vi "Test Resume Refreshing Trigger Broadcast.vi"(8 "error in (no error)":errorcluster, 11 "Test Case In":refnum<class "Debugger Test.lvclass">) -> (0 "error out":errorcluster, 3 "Test Case Out":refnum<class "Debugger Test.lvclass">)   [LabVIEW 2020, in "Debugger Test.lvclass"]
uses:
  Debugger Test.lvclass
  Debugger Test.lvclass/Debugger Test.ctl
  01074fa8-ee8a-411d-bc8b-fc92c4f90959.vi
  source/Process/Debug Process.lvclass
  source/Debugger/Debugger.lvclass
  C:/Git/astemes-triarc-debugger/source/Process/Debug Process.lvclass
  C:/Git/astemes-triarc-debugger/source/Debugger/Debugger.lvclass
  C:/Git/astemes-triarc-debugger/source/Debug Data Event/Debug Data Listener.lvclass
  <vilib>/Astemes/Triarc Framework/Broadcast Event Helpers/Broadcast Event Helpers.lvlib
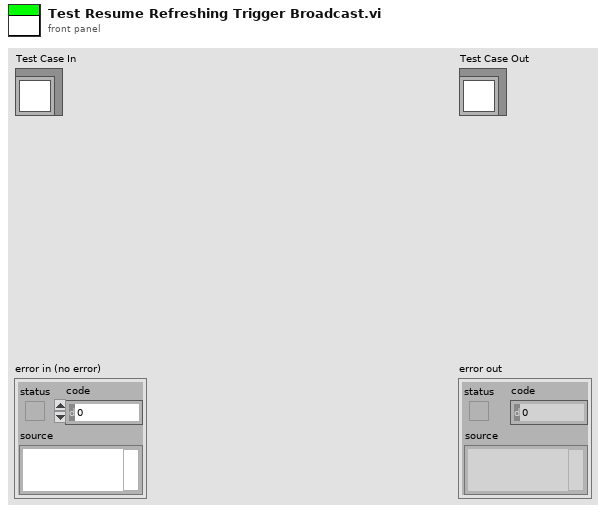
[diagram p1: front panel]
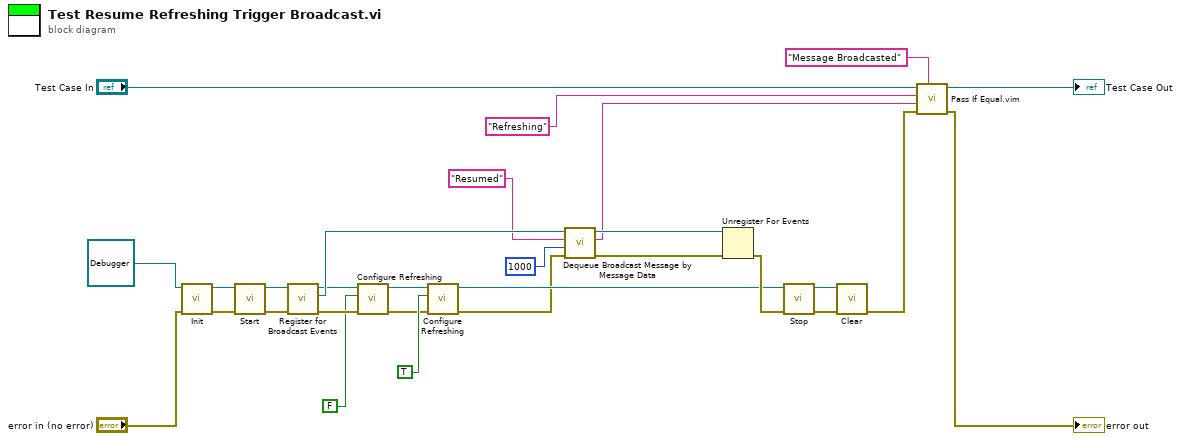
[diagram p0: block diagram]
diagram:
  n1 = call-dynamic "Init.vi"("error in (no error)"="error in (no error)", "Process In"=refnum<class "Debugger.lvclass"> refnum ("Debug Data Event In 2")) -> ("error out"=w25:errorcluster, "Process Out"=w26:refnum<class "Debugger.lvclass">)  [unwired: 8 in]
  n2 = call "Start.vi"("error in (no error)"=w25, "Process In"=w26) -> ("error out"=w23:errorcluster, "Process Out"=w24:refnum<class "Debugger.lvclass">)  [unwired: 7 in, 1 out]
  n3 = call "Register for Broadcast Events.vi"("error in (no error)"=w23, "Process In"=w24) -> ("error out"=w15:errorcluster, "Event Registration Refnum Out"=w16:refnum<event-registration>, "Process Out"=w6:refnum<class "Debugger.lvclass">)  [unwired: 7 in]
  n4 = call "Configure Refreshing.vi"("error in (no error)"=w15, "Refresh?"=FALSE, "Debugger In"=w6) -> ("error out"=w7:errorcluster, "Debugger Out"=w5:refnum<class "Debugger.lvclass">)  [unwired: 7 in]
  n5 = call "Configure Refreshing.vi"("error in (no error)"=w7, "Refresh?"=TRUE ("Show Send?"), "Debugger In"=w5) -> ("error out"=w8:errorcluster, "Debugger Out"=w9:refnum<class "Debugger.lvclass">)  [unwired: 7 in]
  n6 = call <vilib>:"Dequeue Broadcast Message by Message Data.vi"("error in (no error)"=w8, "Timeout (-1)"=1000, "Message Data"="Resumed" ("Message"), "Event Registration Refnum"=w16) -> ("error out"=w10:errorcluster, "Message"=w3:string, "Event Registration Refnum Out"=w12:refnum<event-registration>)  [unwired: 3 in, 2 out]
  n7 = Unregister For Events(event registration refnum=w12, error in=w10) -> (error out=w14:errorcluster)
  n8 = call "Stop.vi"("error in (no error)"=w14, "Process In"=w9) -> ("error out"=w21:errorcluster, "Process Out"=w22:refnum<class "Debugger.lvclass">)  [unwired: 7 in, 1 out]
  n9 = call-dynamic "Clear.vi"("error in (no error)"=w21, "Process In"=w22) -> ("error out"=w18:errorcluster)  [unwired: 9 in]
  n10 = call "Pass If Equal.vim"("Description"="Message Broadcasted", "error in (no error)"=w18, "Actual"=w3, "Expected"="Refreshing" ("Message"), "LUnit Test Case In"="Test Case In") -> ("error out"=→"error out":errorcluster, "LUnit Test Case Out"=→"Test Case Out":refnum<class "Debugger Test.lvclass">)  [unwired: 5 in]
